vi "remove channel test.vi"() -> ()   [LabVIEW 2013, in "sample module tests.lvlib"]
uses:
  sample module tests.lvlib
  module/configuration/sample module configuration.lvclass
panel:
  out "no err":errorcluster
  out "channels match":bool
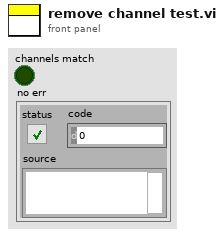
[diagram p1: front panel]
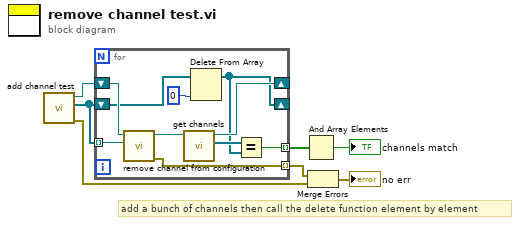
[diagram p0: block diagram]
diagram:
  # "add a bunch of channels then call the delete function element by element"
  n1 = call "add channel test.vi"() -> ("no error"=w1:errorcluster, "channels"=w2:refnum<class "TBM channel.lvclass">[], "sample module configuration out"=w3:refnum<class "sample module configuration.lvclass">)  [unwired: 8 in, 1 out]
  n2 = for {
    shift-right: [w12] -> _
    shift-left: w3 -> [w17]
    tunnel: w2 -> [w16] mode=indexing
    tunnel: [w11] -> w6 mode=indexing
    tunnel: [w9] -> w5 mode=indexing
    shift-right: [w8] -> _
    shift-left: w2 -> [w15]
    n3 = call "remove channel from configuration.vi"("channel"=w16, "sample module configuration in"=w17) -> ("error out"=w11:errorcluster, "sample module configuration out"=w13:refnum<class "sample module configuration.lvclass">)  [unwired: 8 in]
    n4 = call-dynamic "get channels.vi"("module configuration in"=w13) -> ("channels"=w10:refnum<class "TBM channel.lvclass">[], "module configuration out"=w12:refnum<class "sample module configuration.lvclass">)  [unwired: 9 in]
    n5 = Delete From Array(array=w15, index=0) -> (array with subset deleted=w8:refnum<class "TBM channel.lvclass">[])  [unwired: 1 in, 1 out]
    n6 = Equal?(x=w10, y=w8) -> (x = y?=w9:bool)
  }
  n7 = And Array Elements(Boolean array=w5) -> (logical AND=→"channels match":bool)
  n8 = Merge Errors(w6, w1) -> (→"no err":errorcluster)
